vi "Calculate_Triggers_1_Channel.vi"(11 "ChanSettings":T1) -> (1 "Low":fxp<+/-,18,5>, 2 "High":fxp<+/-,18,5>, 3 "WindowTrig":T2)   [LabVIEW 2021]
uses:
  Controls/Clust/WindowTriggerClust.ctl
  <instrlib>/_niInstr/Data Trigger/v1/Shared/Public/Level Configuration FXP(+-,18,1).ctl
  <instrlib>/_niInstr/Data Trigger/v1/Shared/Public/Level Configuration Trigger When.ctl
  Host/Clusts/ChannelWindowClust.ctl
  <vilib>/rvi/FXPMathLib/FxpSub/XNode/nifxpmath_Sub.xnode
  <vilib>/rvi/FXPMathLib/FxpAdd/XNode/nifxpmath_Add.xnode
  <instrlib>/_niInstr/Data Trigger/v1/Shared/niInstr Data Trigger v1 Shared.lvlib
  <vilib>/rvi/FXPMathLib/sim/FxpSim.dll
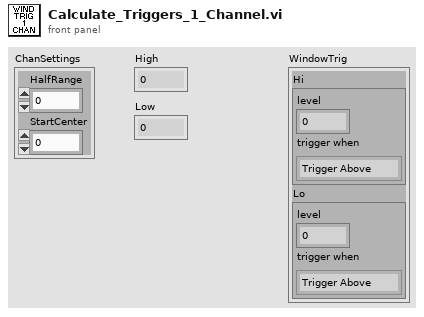
[diagram p1: front panel]
types:
  T1 = typedef "ChannelWindowClust.ctl" = cluster{"HalfRange":fxp<+/-,18,5>, "StartCenter":fxp<+/-,18,5>}
  T2 = typedef "WindowTriggerClust.ctl" = cluster{"Hi":T3, "Lo":T3}
  T3 = typedef "niInstr Data Trigger v1 Shared.lvlib/Level Configuration FXP(+-,18,1).ctl" = cluster{"level":fxp<+/-,18,5>, "trigger when":T4}
  T4 = typedef "niInstr Data Trigger v1 Shared.lvlib/Level Configuration Trigger When.ctl" = enum8{"Trigger Above", "Trigger Below"}
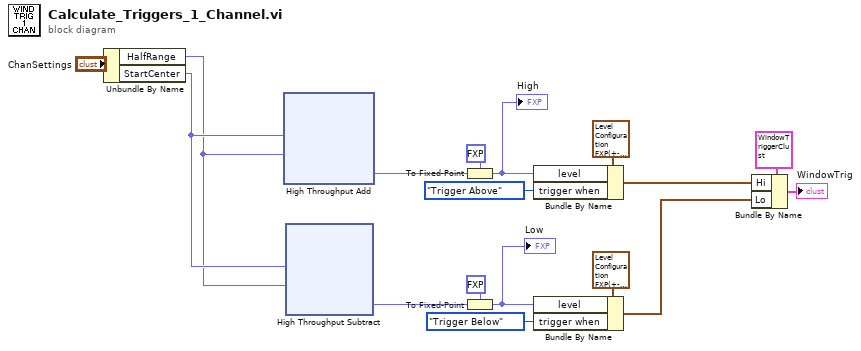
[diagram p0: block diagram]
diagram:
  n1 = Unbundle By Name("ChanSettings") -> ("HalfRange"=w1:fxp<+/-,18,5>, "StartCenter"=w3:fxp<+/-,18,5>)
  n2 = xnode ("High Throughput Add")("x"=w3, "y"=w1) -> ("x+y"=w5:fxp<+/-,19,6>)
  n3 = xnode ("High Throughput Subtract")("x"=w3, "y"=w1) -> ("x-y"=w11:fxp<+/-,19,6>)
  n4 = To Fixed-Point(fixed-point type=fxp<+/-,18,5> 0.0 ("StartCenter"), number=w5) -> (fixed-point=w7:fxp<+/-,18,5>)
  "High" <- w7
  n5 = To Fixed-Point(fixed-point type=fxp<+/-,18,5> 0.0 ("StartCenter"), number=w11) -> (fixed-point=w12:fxp<+/-,18,5>)
  "Low" <- w12
  n6 = Bundle By Name(cluster=T3 {"level"=0.0, "trigger when"=enum."Trigger Above"} ("trigger.level"), "level"=w7, "trigger when"=Level_Configuration_Trigger_When."Trigger Above") -> (w15:T3)
  n7 = Bundle By Name(cluster=T3 {"level"=0.0, "trigger when"=enum."Trigger Above"} ("trigger.level"), "level"=w12, "trigger when"=Level_Configuration_Trigger_When."Trigger Below") -> (w16:T3)
  n8 = Bundle By Name(cluster=T2 {"Hi"={"level"=0.0, "trigger when"=enum."Trigger Above"}, "Lo"={"level"=0.0, "trigger when"=enum."Trigger Above"}}, "Hi"=w15, "Lo"=w16) -> (→"WindowTrig":T2)
